vi "OBJ_parse_result_save_response.vi"(8 "error_in":errorcluster, 9 "measurement_right":string, 10 "measurement_left":string, 11 "sql_results_in":variant) -> (0 "error_out":errorcluster, 4 "test_ok?":bool)   [LabVIEW 2019]
uses:
  FGV/tristate_indicator_OBJ_test/FGV_tristate_indicator_OBJ_test.ctl
  FGV/test_button/FGV_OBJ_test_button.ctl
  FGV/OBJ_records_display/FGV_OBJ_records_display.ctl
  <vilib>/addons/database/_DB Variant To Data/Database Variant To Data.xnode
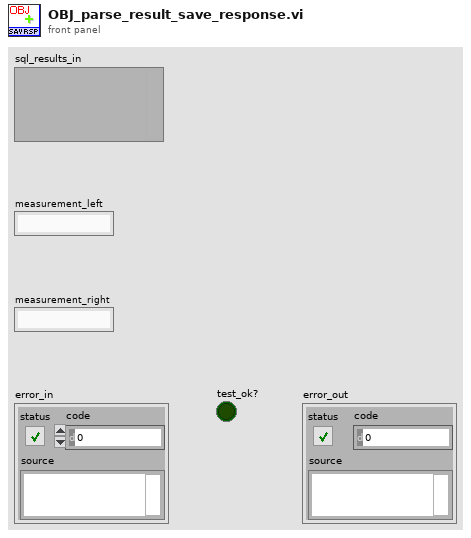
[diagram p1: front panel]
types:
  T1 = typedef "FGV_OBJ_test_button.ctl" = enum16{"initialize", "set_new_login", "set_message", "enable", "disable", "disable_gray", "translate"}
  T2 = typedef "FGV_tristate_indicator_OBJ_test.ctl" = enum16{"initialize", "ready", "pending", "OK", "NOK", "part_NOK", "routing_NOK", "repeat_NOK", "timeout", "translate", "error"}
  T3 = typedef "FGV_OBJ_records_display.ctl" = enum16{"initialize", "set_serial", "display_header", "display_results", "get_serial", "get_part_ID", "clear"}
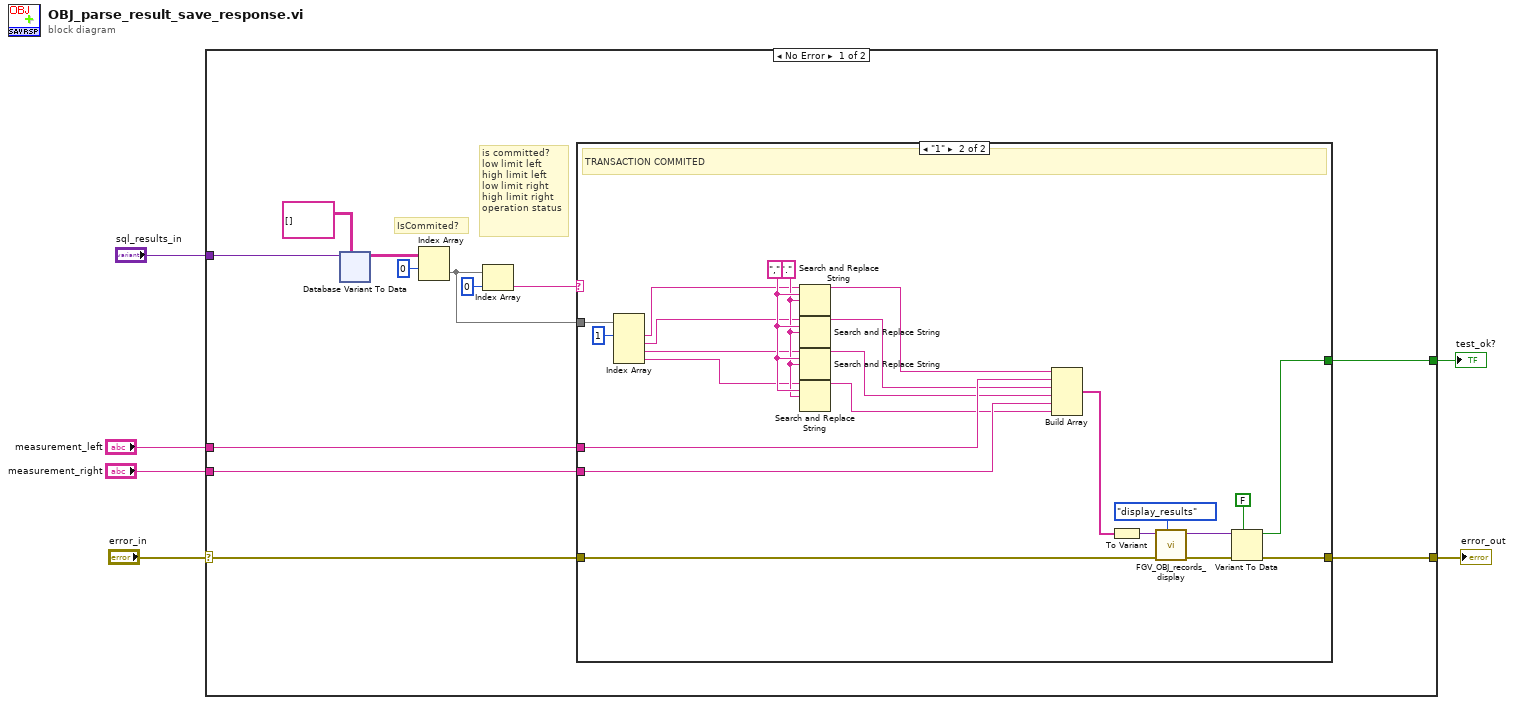
[diagram p0: block diagram]
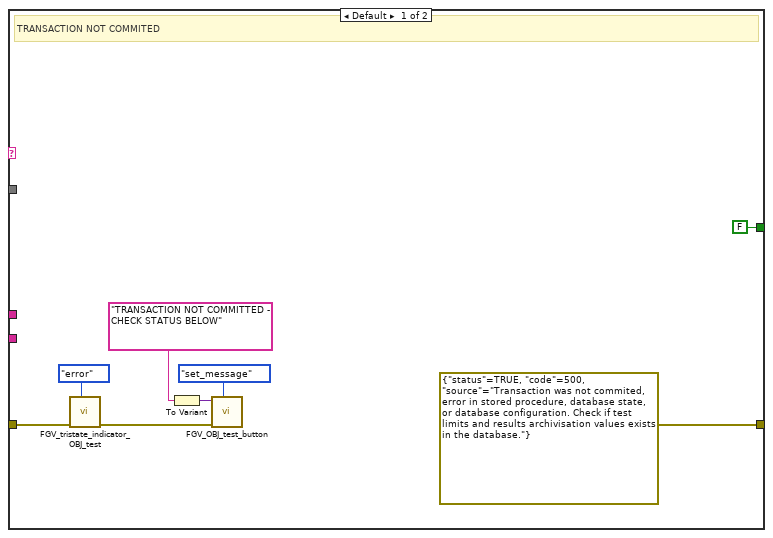
[diagram p2: hidden frame]
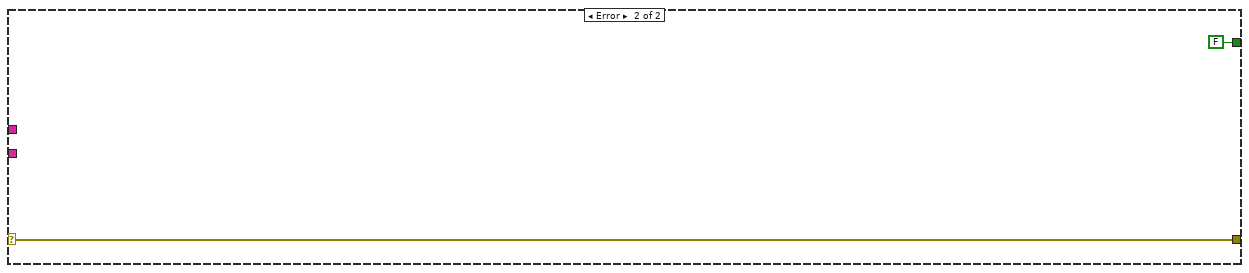
[diagram p3: hidden frame]
diagram:
  n1 = case shown="No Error" "error_in" {
    selector: "error_in" -> [w16 w83]
    tunnel: "sql_results_in" -> [w13 _]
    tunnel: [w15 w83] -> w5
    tunnel: "measurement_left" -> [w10 _]
    tunnel: "measurement_right" -> [w9 _]
    tunnel: [w7 FALSE] -> w1
    frame No Error {
      # "is committed?\nlow limit left\nhigh limit left\nlow limit right\nhigh limit right\noperation status"
      # "IsCommited?"
      n2 = xnode "Database Variant To Data"("database variant"=w13, "type"=string[][] []) -> ("data"=w17:string[][])  [unwired: 1 in, 1 out]
      n3 = Index Array(array=w17, index (row)=0) -> (element=w8:string[])  [unwired: 1 in]
      n4 = Index Array(array=w8, index=0) -> (element=w11:string)
      n5 = case shown="\"1\"" w11 {
        tunnel: w16 -> [w53 w80]
        tunnel: [errorcluster {"status"=TRUE, "code"=500, "source"="Transaction was not commited, error in stored procedure, database state, or database configuration. Check if test limits and results archivisation values exists in the database."} ("error IO") w70] -> w15
        tunnel: w10 -> [_ w75]
        tunnel: w9 -> [_ w74]
        tunnel: w8 -> [_ w77]
        tunnel: [FALSE w69] -> w7
        frame Default {
          # "TRANSACTION NOT COMMITED"
          n6 = call "FGV_tristate_indicator_OBJ_test.vi"("options"=FGV_tristate_indicator_OBJ_test."error", "error_in"=w53) -> ("error_out"=w52:errorcluster)  [unwired: 9 in]
          n7 = To Variant(anything="TRANSACTION NOT COMMITTED - CHECK STATUS BELOW") -> (Variant=w55:variant)
          n8 = call "FGV_OBJ_test_button.vi"("options"=FGV_OBJ_test_button."set_message", "error_in"=w52, "input"=w55) -> ()  [unwired: 8 in, 1 out]
        }
        frame "1" {
          w67 = "." ("replace string (\"\")")
          w68 = "," ("search string")
          # "TRANSACTION COMMITED"
          n9 = Index Array(array=w77, index #1=1 ("index")) -> (element #1=w66:string, element #2=w64:string, element #3=w62:string, element #4=w60:string)  [unwired: 3 in]
          n10 = Search and Replace String(input string=w66, search string=w68, replace string=w67) -> (result string=w65:string)  [unwired: 5 in, 3 out]
          n11 = Search and Replace String(input string=w64, search string=w68, replace string=w67) -> (result string=w63:string)  [unwired: 5 in, 3 out]
          n12 = Search and Replace String(input string=w62, search string=w68, replace string=w67) -> (result string=w61:string)  [unwired: 5 in, 3 out]
          n13 = Search and Replace String(input string=w60, search string=w68, replace string=w67) -> (result string=w59:string)  [unwired: 5 in, 3 out]
          n14 = Build Array(w65, w75, w63, w61, w74, w59) -> (w78:string[])
          n15 = To Variant(anything=w78) -> (Variant=w79:variant)
          n16 = call "FGV_OBJ_records_display.vi"("options"=FGV_OBJ_records_display."display_results", "error_in"=w80, "input"=w79) -> ("error_out"=w71:errorcluster, "output"=w72:variant)  [unwired: 7 in]
          n17 = Variant To Data(error in=w71, type=FALSE, Variant=w72) -> (data=w69:bool, error out=w70:errorcluster)
        }
      }
    }
    frame Error {
    }
  }
  "error_out" <- w5
  "test_ok?" <- w1
